vi "Initialise.vi"(8 "error in (no error)":errorcluster, 11 "Process":refnum<vi>) -> (0 "error out":errorcluster, 3 "Actor out":refnum<class "System Status Actor.lvclass">, 5 "Mailboxes":cluster{"Mailbox":refnum<event-registration>})   [LabVIEW 2020, in "RTAF.lvlib" / "System Status Actor.lvclass"]
uses:
  System Status Actor.lvclass
  C:/dev/PGS/2001 - TBCM/Source/RT/RTAF/Source/RTAF/Actors/Base Actor/Actor/Actor.lvclass
  Base Actor/Actor/Message.ctl
  System Status Actor.lvclass/System Status Actor.ctl
  Global References.vi
  Base Actor/API/Actor API.lvclass
  Base Actor/Actor/Actor.lvclass
  RTAF.lvlib
  API/System Status Actor API.lvclass
  C:/dev/PGS/2001 - TBCM/Source/RT/RTAF/Source/RTAF/Actors/System Status/Actor/System Status Actor.lvclass
  C:/dev/PGS/2001 - TBCM/Source/RT/RTAF/Source/RTAF/Actors/Base Actor/API/Actor API.lvclass
  C:/dev/PGS/2001 - TBCM/Source/RT/RTAF/Source/RTAF/Actors/System Status/API/System Status Actor API.lvclass
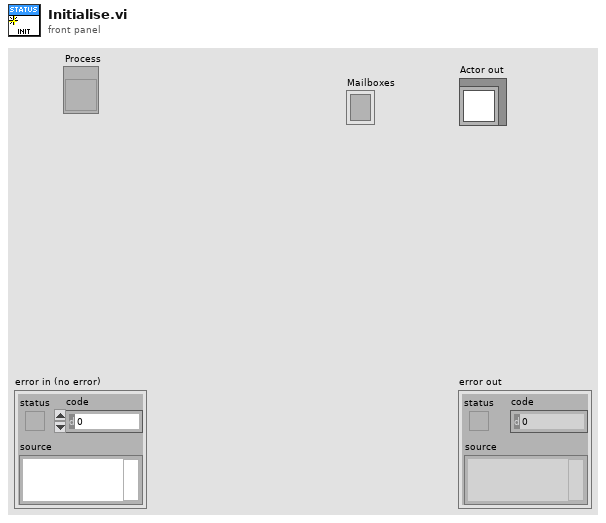
[diagram p1: front panel]
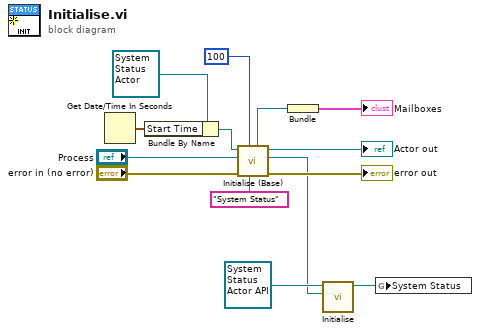
[diagram p0: block diagram]
diagram:
  n1 = Get Date/Time In Seconds() -> (seconds since 1Jan1904=w1:timestamp)
  n2 = Bundle By Name(cluster=refnum<class "System Status Actor.lvclass"> refnum ("Test Actor.lvclass"), "Start Time"=w1) -> (w2:refnum<class "System Status Actor.lvclass">)
  n3 = call "Initialise (Base).vi"("Name"="System Status", "Tick Period [100 ms]"=100, "error in (no error)"="error in (no error)", "Process"="Process", "Actor in"=w2) -> ("error out"=→"error out":errorcluster, "Message Channel"=w9:refnum<user-event>, "Actor out"=→"Actor out":refnum<class "System Status Actor.lvclass">, "Mailbox"=w4:refnum<event-registration>)  [unwired: 3 in]
  n4 = Bundle("Mailbox"=w4) -> (→"Mailboxes":cluster{"Mailbox":refnum<event-registration>})  [unwired: 1 in]
  n5 = call "Initialise.vi"("Message Channel"=w9, "Actor API in"=refnum<class "System Status Actor API.lvclass"> refnum ("Test Actor API.lvclass")) -> ("Actor API out"=w7:refnum<class "System Status Actor API.lvclass">)  [unwired: 9 in]
  n6 = global write "Global References.vi" "System Status"(w7) -> ()
